vi "Diconnect from library.vi"() -> ()   [LabVIEW 2012]
panel:
  out "Out Of...":i32
  out "File":i32
  out "Path":path
  in  "vi base path":path=path "C:/perforce/Regression/Automation/LabVIEW"
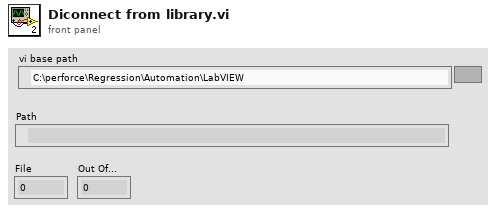
[diagram p1: front panel]
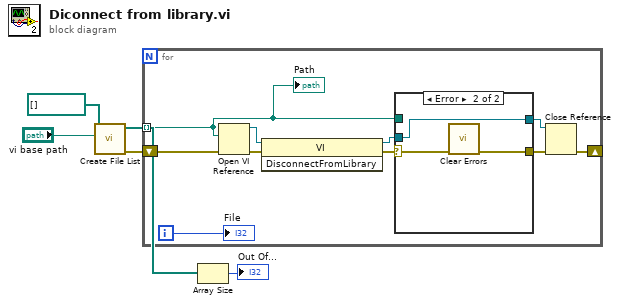
[diagram p0: block diagram]
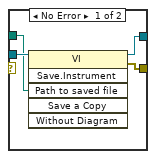
[diagram p2: hidden frame]
diagram:
  n1 = call "Create File List.vi"("vi base path"="vi base path", "File Path Array in"=path[] []) -> ("error out"=w4:errorcluster, "File Path Array out"=w3:path[])  [unwired: 8 in]
  n2 = for {
    tunnel: w3 -> [w6] mode=indexing
    shift-right: [w8] -> _
    shift-left: w4 -> [w15]
    i -> [w7]
    n3 = Open VI Reference(vi path=w6, error in (no error)=w15) -> (vi reference=w14:refnum<vi>, error out=w13:errorcluster)  [unwired: 4 in]
    n4 = invoke class="VI" method="DisconnectFromLibrary"(reference=w14, error in=w13) -> (reference out=w10:refnum<vi>, error out=w12:errorcluster)  [unwired: 1 in, 1 out]
    n5 = case shown="Error" w12 {
      selector: w12 -> [_ w22]
      tunnel: [w16 w21] -> w11
      tunnel: w10 -> [w19 w20]
      tunnel: w6 -> [w18 _]
      tunnel: [w17 w20] -> w9
      frame No Error {
        n6 = invoke class="VI" method="Save.Instrument"(reference=w19, "Path to saved file"=w18) -> (reference out=w17:refnum<vi>, error out=w16:errorcluster)  [unwired: 4 in, 4 out]
      }
      frame Error {
        n7 = call <vilib>:"Clear Errors.vi"("error in (no error)"=w22) -> ("error out"=w21:errorcluster)  [unwired: 6 in]
      }
    }
    n8 = Close Reference(reference=w9, error in (no error)=w11) -> (error out=w8:errorcluster)
    "Path" <- w6
    "File" <- w7
  }
  n9 = Array Size(array=w3) -> (size(s)=→"Out Of...":i32)
